vi "Get Number of Impulses.vi"(8 "error in (no error)":errorcluster, 11 "Impulse Manager in":refnum<class "Impulse Manager.lvclass">) -> (0 "error out":errorcluster, 2 "Number of impulses":i32, 3 "Impulse Manager out":refnum<class "Impulse Manager.lvclass">)   [LabVIEW 2016, in "Impulse Manager.lvclass"]
uses:
  Impulse Manager.lvclass
  Impulse Manager.lvclass/Impulse Manager.ctl
  Impulse Data/Impulse Data.lvclass
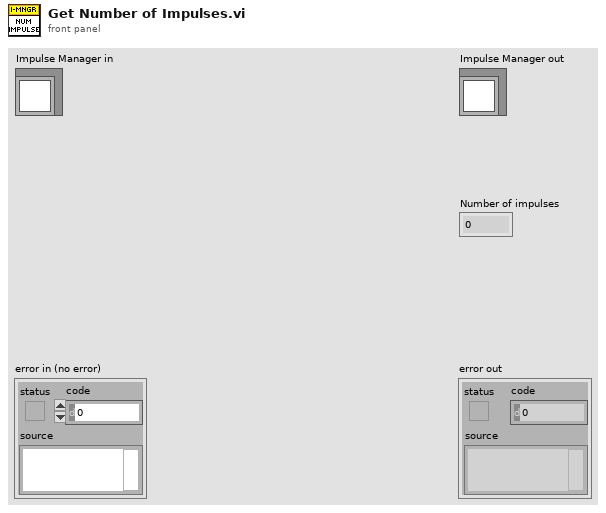
[diagram p1: front panel]
types:
  T1 = typedef "Impulse Data.lvclass/Instance handle.ctl" = refnum<data-value>
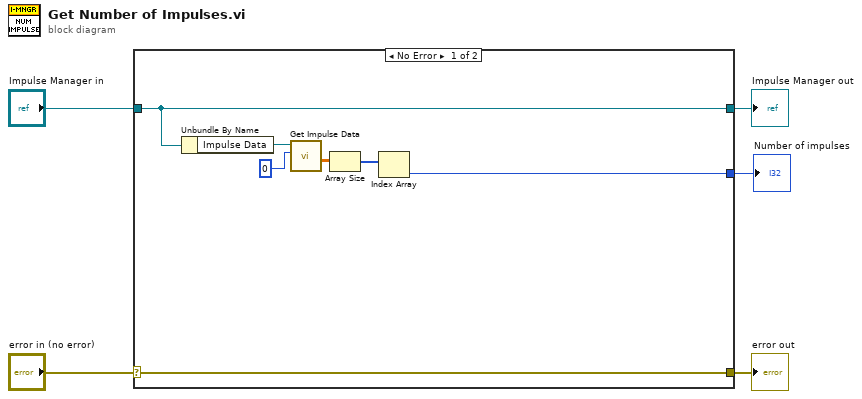
[diagram p0: block diagram]
diagram:
  n1 = case shown="No Error" "error in (no error)" {
    selector: "error in (no error)" -> [w12 w14]
    tunnel: [w12 w14] -> w4
    tunnel: [w11 w13] -> w2
    tunnel: "Impulse Manager in" -> [w11 w13]
    tunnel: [w6 _] -> w1
    frame No Error {
      n2 = Unbundle By Name(w11) -> ("Impulse Data"=w10:T1)
      n3 = call "Get Impulse Data.vi"("Channel"=0, "Reference in"=w10) -> ("Impulses out"=w8:dbl[][])  [unwired: 8 in, 1 out]
      n4 = Array Size(array=w8) -> (size(s)=w7:i32[])
      n5 = Index Array(array=w7) -> (element=w6:i32)  [unwired: 1 in]
    }
    frame Error {
    }
  }
  "error out" <- w4
  "Impulse Manager out" <- w2
  "Number of impulses" <- w1
